vi "Next_Temp.vi"(7 "Temp and Field Range in":T1, 8 "error in (no error)":errorcluster, 9 "Field and Temp Array Controller":cluster{"Field (T)":dbl[], "Temps (K)":dbl[]}, 10 "SweepQ in":refnum<queue>, 11 "Queue in":refnum<queue>) -> (0 "error out":errorcluster, 1 "Temp and Field Range out":T1, 2 "SweepQ out":refnum<queue>, 3 "Queue out":refnum<queue>)   [LabVIEW 2025]
uses:
  CTLS/TC-Cluster.ctl
  <userlib>/Nanonis Prog Interface V5e/Nanonis Prog Interface.lvlib
  CTLS/Sweeper.ctl
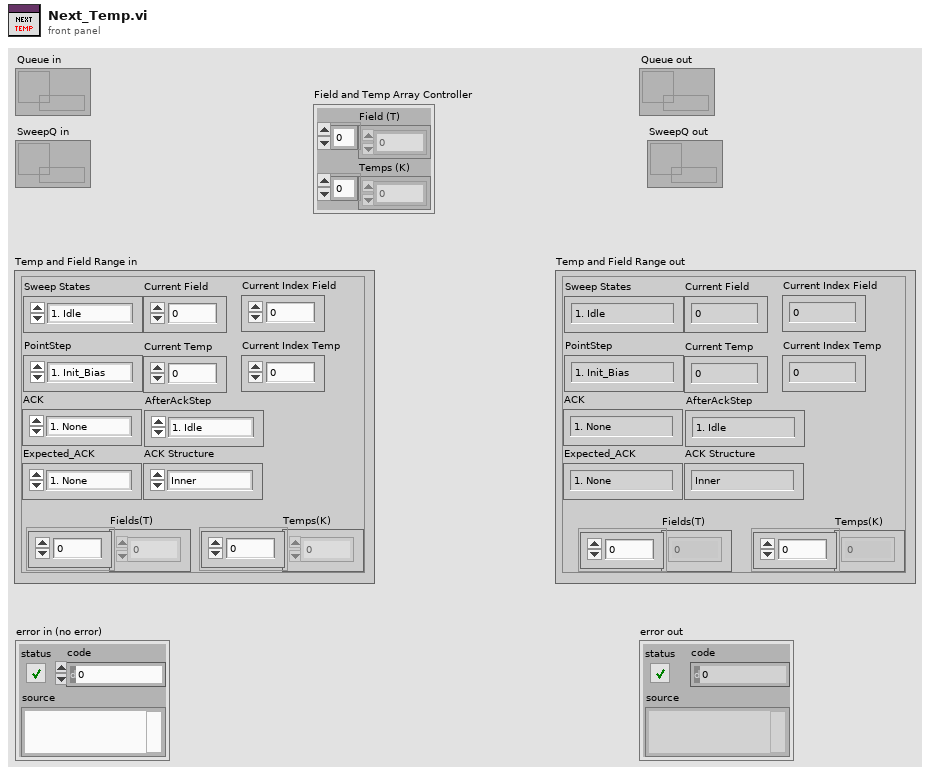
[diagram p1: front panel]
types:
  T1 = typedef "Sweeper.ctl" = cluster{"Temps(K)":dbl[], "Fields(T)":dbl[], "Sweep States":enum16{"1. Idle", "2. Start", "3. Apply_Config", "4. Run_Point_Step", "5. Wait ACK", "6. Next Field", "7. Next Temp", "8. Stop"}, "PointStep":enum16{"1. Init_Bias", "2. Init_Scan", "3. Field_Stable", "4. Temp_stable", "1. Scan_1", "2. DC_SF_1", "3. DC_BS_1", "4. Bias", "5. Scan_2", "6. DC_SF_2", "7. DC_BS_2", "8. Done"}, "Current Field":dbl, "Current Temp":dbl, "Expected_ACK":enum16{"1. None", "2. TempStable", "3. FieldStable", "4. ConfigApplied", "5. ScanDone", "6. BiasDone", "7. DriftDone (SF)", "8. DrifDone (BS)", "9. Done"}, "ACK":enum16{"1. None", "2. TempStable", "3. FieldStable", "4. ConfigApplied", "5. ScanDone", "6. BiasDone", "7. DriftDone (SF)", "8. DrifDone (BS)", "9. Done"}, "AfterAckStep":enum16{"1. Idle", "2. Start", "3. Apply_Config", "4. Run_Point_Step", "5. Wait ACK", "6. Next Field", "7. Next Temp", "8. Stop"}, "Current Index Field":i32, "Current Index Temp":i32, "ACK Structure ":enum16{"Inner", "Outer"}}
  T2 = enum16{"1. INIT TEMP", "2. TC ON", "3. TEMP_STAB", "4. TC IDLE", "5. TC OFF (Reset)"}
  T3 = typedef "TC-Cluster.ctl" = cluster{"Range (0:Off)":u16, "Manual Output (0.00 %)":dbl, "Rate (D) (0.0 %)":dbl, "Reset (I) (20.0)":dbl, "Gain (P) (50.0)":dbl, "Power Up Enable (F: Disable)":bool, "Max User Current (2.000)":dbl, "Heater Resistance (1:25 Ohms)":u16, "Max Current (0:User Specified)":u16, "Heater Out Display (1:Current)":u16, "Mode (0:Off)":u16, "Input (0:None)":u16, "Target Temp (K)":dbl, "Serial Configuration":cluster{"Baud Rate":u32, "Parity":u16, "Data Bits":u16, "Stop Bits":u16, "Flow Control":u16}, "VISA resource name":refnum<visa-resource-name>, "Configure Control Parameters (0: Configure)":u16, "Enable Setpoint (F:Disable)":bool, "Input (0:A)":u16, "Data Source (0:Kelvin)":u16, "Output's Control Loop (1:1)":u16, "STND DEV Threshold ":dbl, "Mean Tolerance ":dbl, "Current State":enum16{"1. INIT TEMP", "2. TC ON", "3. TEMP_STAB", "4. TC IDLE", "5. TC OFF (Reset)"}}
  T4 = enum16{"1. Init_Bias", "2. Init_Scan", "3. Field_Stable", "4. Temp_stable", "1. Scan_1", "2. DC_SF_1", "3. DC_BS_1", "4. Bias", "5. Scan_2", "6. DC_SF_2", "7. DC_BS_2", "8. Done"}
  T5 = enum16{"1. Idle", "2. Start", "3. Apply_Config", "4. Run_Point_Step", "5. Wait ACK", "6. Next Field", "7. Next Temp", "8. Stop"}
  T6 = enum16{"1. None", "2. TempStable", "3. FieldStable", "4. ConfigApplied", "5. ScanDone", "6. BiasDone", "7. DriftDone (SF)", "8. DrifDone (BS)", "9. Done"}
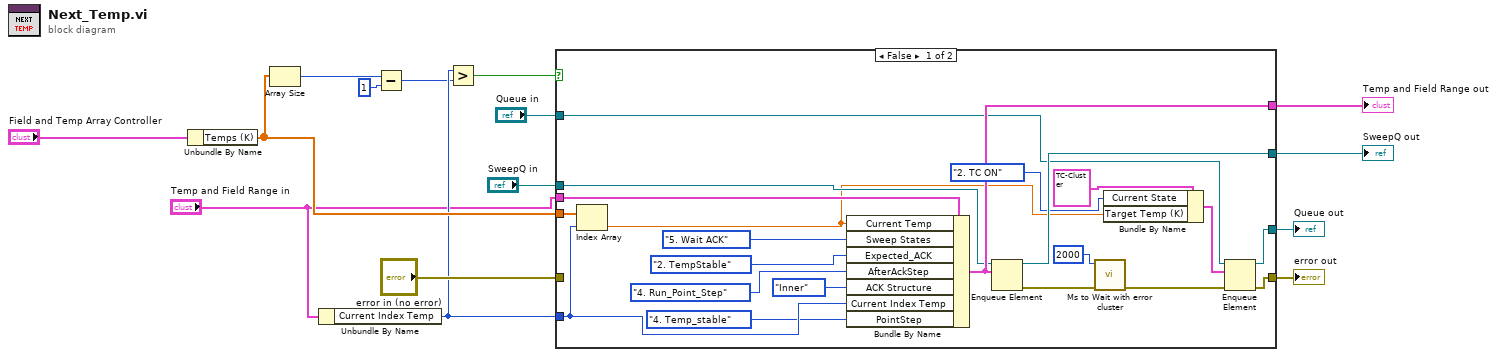
[diagram p0: block diagram]
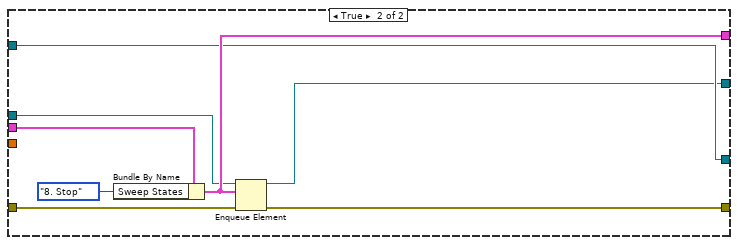
[diagram p2: hidden frame]
diagram:
  n1 = Unbundle By Name("Field and Temp Array Controller") -> ("Temps (K)"=w8:dbl[])
  n2 = Array Size(array=w8) -> (size(s)=w2:i32)
  n3 = Unbundle By Name("Temp and Field Range in") -> ("Current Index Temp"=w7:i32)
  n4 = Subtract(x=w2, y=1 ("x")) -> (x-y=w3:i32)
  n5 = Greater?(x=w7, y=w3) -> (0:w4:bool)
  n6 = case shown="False" w4 {
    tunnel: "Temp and Field Range in" -> [w36 w44]
    tunnel: w7 -> [w30 _]
    tunnel: [w28 w42] -> w6
    tunnel: w8 -> [w31 _]
    tunnel: "SweepQ in" -> [w27 w40]
    tunnel: [w26 w39] -> w11
    tunnel: "Queue in" -> [w22 w41]
    tunnel: [w17 w38] -> w13
    tunnel: [w16 w41] -> w14
    tunnel: "error in (no error)" -> [_ w37]
    frame False {
      n7 = Index Array(array=w31, index=w30) -> (element=w18:dbl)
      n8 = Bundle By Name(cluster=w36, "Current Temp"=w18, "Sweep States"=T5."5. Wait ACK", "Expected_ACK"=T6."2. TempStable", "AfterAckStep"=T5."4. Run_Point_Step", "ACK Structure"=enum16{"Inner", "Outer"}."Inner", "Current Index Temp"=w30, "PointStep"=T4."4. Temp_stable") -> (w28:T1)
      n9 = Enqueue Element(queue=w27, element=w28) -> (queue out=w26:refnum<queue>, error out=w25:errorcluster)  [unwired: 2 in, 1 out]
      n10 = call <userlib>:"Ms to Wait with error cluster.vi"("error in (no error)"=w25, "milliseconds to wait"=u32 2000) -> ("error out"=w23:errorcluster)  [unwired: 4 in, 1 out]
      n11 = Bundle By Name(cluster=T3 {"Range (0:Off)"=0, "Manual Output (0.00 %)"=0.0, "Rate (D) (0.0 %)"=0.0, "Reset (I) (20.0)"=20.0, "Gain (P) (50.0)"=50.0, "Power Up Enable (F: Disable)"=FALSE, "Max User Current (2.000)"=2.0, "Heater Resistance (1:25 Ohms)"=1, "Max Current (0:User Specified)"=0, "Heater Out Display (1:Current)"=1, "Mode (0:Off)"=0, "Input (0:None)"=0, "Target Temp (K)"=0.0, "Serial Configuration"={"Baud Rate"=57600, "Parity"=1, "Data Bits"=7, "Stop Bits"=10, "Flow Control"=0}, "VISA resource name"="", "Configure Control Parameters (0: Configure)"=0, "Enable Setpoint (F:Disable)"=FALSE, "Input (0:A)"=0, "Data Source (0:Kelvin)"=0, "Output's Control Loop (1:1)"=1, "STND DEV Threshold "=0.1, "Mean Tolerance "=0.02, "Current State"=enum."1. INIT TEMP"} ("Temp Controller"), "Current State"=T2."2. TC ON", "Target Temp (K)"=w18) -> (w20:T3)
      n12 = Enqueue Element(queue=w22, element=w20, error in (no error)=w23) -> (queue out=w16:refnum<queue>, error out=w17:errorcluster)  [unwired: 1 in, 1 out]
    }
    frame True {
      n13 = Bundle By Name(cluster=w44, "Sweep States"=T5."8. Stop") -> (w42:T1)
      n14 = Enqueue Element(queue=w40, element=w42, error in (no error)=w37) -> (queue out=w39:refnum<queue>, error out=w38:errorcluster)  [unwired: 1 in, 1 out]
    }
  }
  "Queue out" <- w14
  "error out" <- w13
  "SweepQ out" <- w11
  "Temp and Field Range out" <- w6
